vi "configure_sas.vi"(9 "VISA Refnum in":refnum<visa-resource-name>) -> (0 "error out":errorcluster, 3 "VISA Refnum out":refnum<visa-resource-name>)   [LabVIEW 2019]
uses:
  <instrlib>/Agilent E4360/Agilent E4360.lvlib
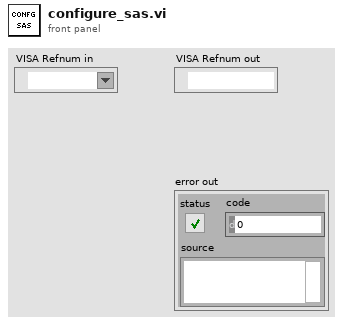
[diagram p1: front panel]
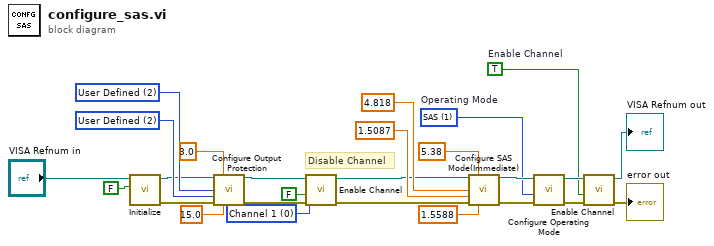
[diagram p0: block diagram]
diagram:
  w1 = 0 items=["Channel 1", "Channel 2", "Channel 1 & Channel 2"] ("Channel List (0:Channel 1)")
  w11 = 2 items=["MAX", "MIN", "User Defined"] ("Voltage Limit Source (0:MAX)")
  w10 = 2 items=["MAX", "MIN", "User Defined"] ("Current Limit Source (0:MAX)")
  w5 = TRUE  # Enable Channel
  w4 = 1 items=["Fixed", "SAS", "Table"]  # Operating Mode
  # "Disable Channel"
  n1 = call <instrlib>:"Initialize.vi"("ID Query (True)"=FALSE, "VISA resource name"="VISA Refnum in") -> ("error out"=w7:errorcluster, "VISA resource name out"=w6:refnum<visa-resource-name>)  [unwired: 8 in]
  n2 = call <instrlib>:"Configure Output Protection.vi"("VISA resource name"=w6, "Current Limit (0 A)"=3.0, "Current Limit Source (0:MAX)"=w10, "Voltage Limit Source (0:MAX)"=w11, "error in (no error)"=w7, "Voltage Limit (0 V)"=15.0) -> ("VISA resource name out"=w20:refnum<visa-resource-name>, "error out"=w21:errorcluster)  [unwired: 8 in]
  n3 = call <instrlib>:"Enable Channel.vi"("error in (no error)"=w21, "Enable Channel (Disable)"=FALSE, "Channel List (0:Channel 1)"=w1, "VISA resource name"=w20) -> ("error out"=w13:errorcluster, "VISA resource name out"=w12:refnum<visa-resource-name>)  [unwired: 6 in]
  n4 = call <instrlib>:"Configure SAS Mode(Immediate).vi"("VISA resource name"=w12, "Open Circuit Voltage (0.0 V)"=5.38, "Maximum Voltage Point (0.0 V)"=4.818, "Maximum Current Point (0.0 A)"=1.5087, "error in (no error)"=w13, "Short Circuit Current (0.0 A)"=1.5588) -> ("VISA resource name out"=w18:refnum<visa-resource-name>, "error out"=w19:errorcluster)  [unwired: 8 in]
  n5 = call <instrlib>:"Configure Operating Mode.vi"("error in (no error)"=w19, "Operating Mode (0:Fixed)"=w4, "VISA resource name"=w18) -> ("error out"=w23:errorcluster, "VISA resource name out"=w22:refnum<visa-resource-name>)  [unwired: 7 in]
  n6 = call <instrlib>:"Enable Channel.vi"("error in (no error)"=w23, "Enable Channel (Disable)"=w5, "VISA resource name"=w22) -> ("error out"=→"error out":errorcluster, "VISA resource name out"=→"VISA Refnum out":refnum<visa-resource-name>)  [unwired: 7 in]
